vi "cRIO_PBP.vi"() -> ()   [LabVIEW 2013]
panel:
  out "SGFref1":u32=100000000
  in  "SGSignalType1":u8
  in  "SGUpdateRate1":u32=40
  in  "SGPhase1":u32
  in  "SGFreq1":u32=100000
  in  "SGAmp1":u16=1
  out "SGFref0":u32=100000000
  in  "SGSignalType0":u8
  in  "SGUpdateRate0":u32=40
  in  "SGPhase0":u32
  in  "SGFreq0":u32=100000
  in  "SGAmp0":u16=1
  out "SGNo":u8=2
  out "auxDI1":bool
  out "auxDI0":bool
  out "DI1":bool
  out "DI0":bool
  in  "auxDO1":bool
  in  "auxDO0":bool
  in  "DO1":bool
  in  "DO0":bool
  in  "AOEnable1":bool
  in  "AOEnable0":bool
  in  "auxAO1":i32
  in  "auxAO0":i32
  in  "AO1":i32
  in  "AO0":i32
  out "auxAI1":i32
  out "auxAI0":i32
  out "AI1":i32
  out "AI0":i32
  in  "SamplingRate1":u16=10000
  in  "SamplingRate0":u16=10000
  in  "DebugMode":bool
  in  "DAQStartStop":bool
  out "DevProfile":enum8{"DAQ", "PBP"}(ring)=enum."PBP"
  out "DevTemp":i16=-10244
  out "DevQualityStatus":u8
  out "Fref":u32=100000000
  out "cRIOModulesOK":bool=TRUE
  out "InsertedIOModulesID":u16[](array[numeric])
  out "InitDone":bool=TRUE
  out "FPGAVIversion":u8[](array[numeric])=[1, 0]
  out "Platform":enum8{"FlexRIO", "cRIO", "RSeries"}(ring)=enum."cRIO"
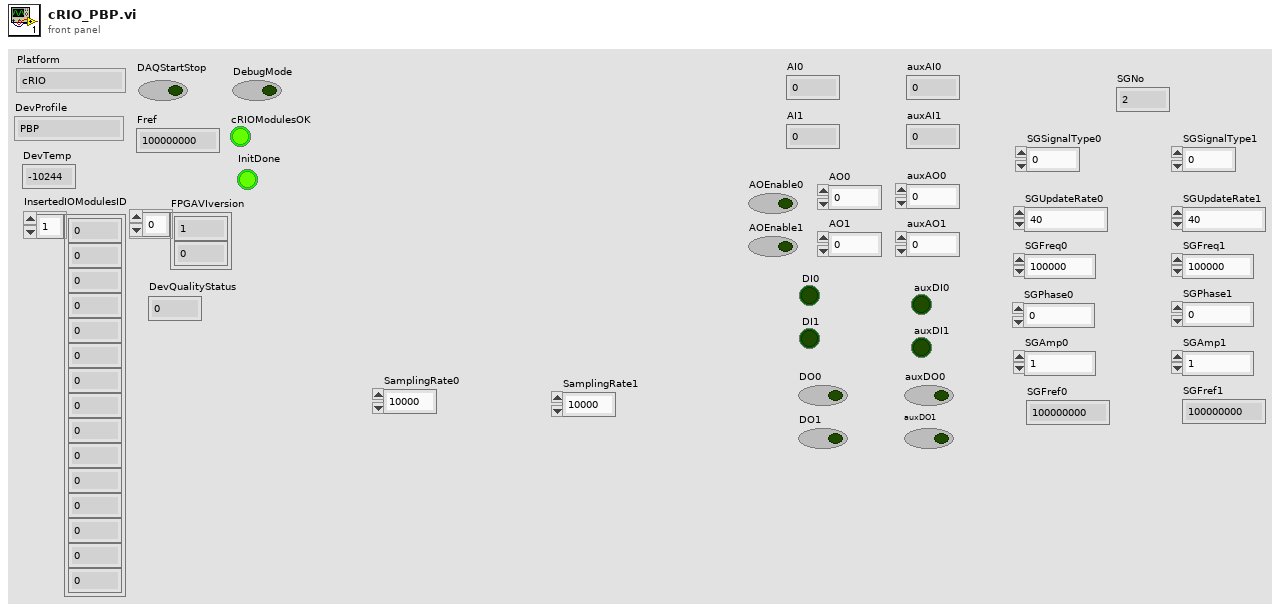
[diagram p1: front panel]
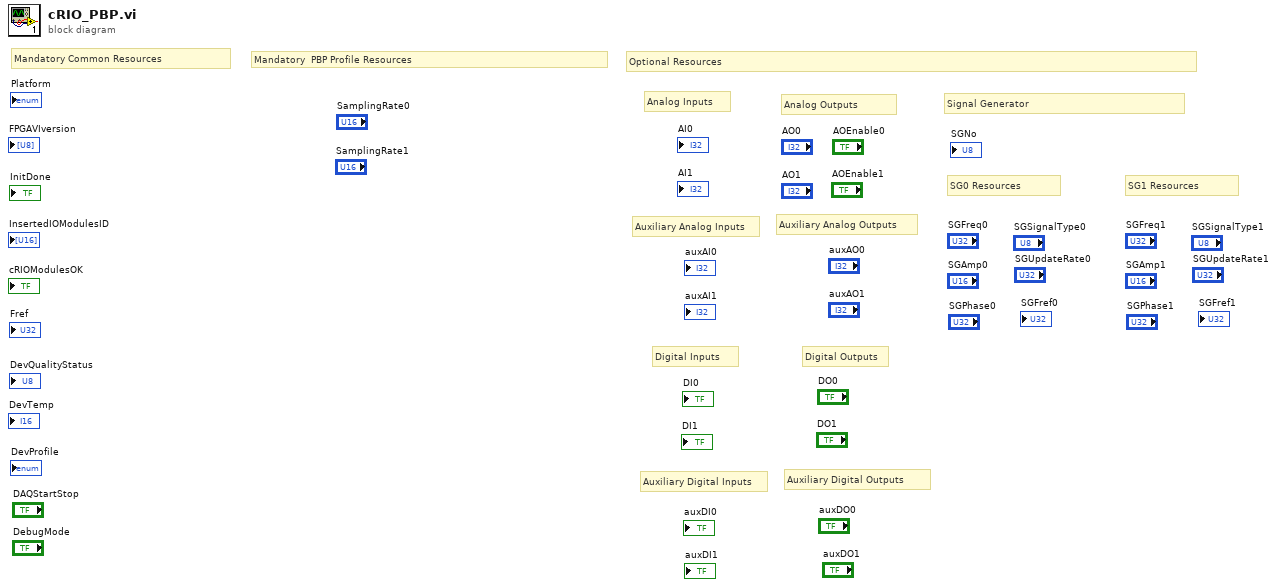
[diagram p0: block diagram]
diagram:
  # "SG1 Resources"
  # "SG0 Resources"
  # "Signal Generator"
  # "Digital Outputs"
  # "Auxiliary Digital Outputs"
  # "Auxiliary Digital Inputs"
  # "Digital Inputs"
  # "Auxiliary Analog Outputs"
  # "Analog Outputs"
  # "Auxiliary Analog Inputs"
  # "Analog Inputs"
  # "Optional Resources"
  # "Mandatory  PBP Profile Resources"
  # "Mandatory Common Resources"
